vi "Set - TFA User Control Refs.vi"(0 "reference in":refnum<class "SPWB.lvclass">, 5 "error in (no error)":errorcluster, 7 "TFA User Control Refs":T1) -> (14 "reference out":refnum<class "SPWB.lvclass">, 19 "error out":errorcluster)   [LabVIEW 2022 SP3, in "SPWB.lvclass"]
uses:
  SPWB.lvclass
  controls/TFA - User Control References.ctl
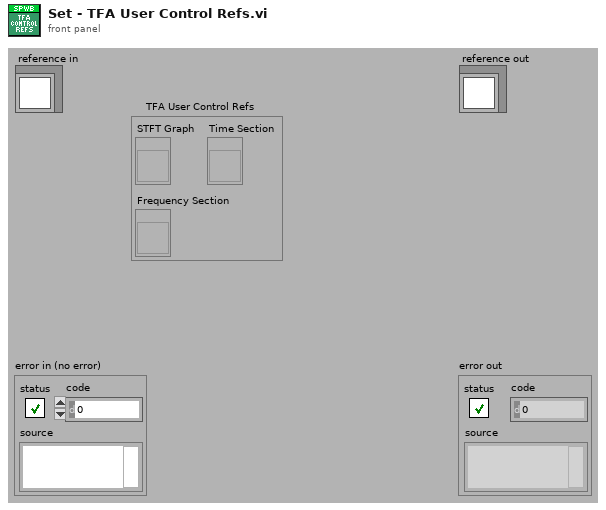
[diagram p1: front panel]
types:
  T1 = typedef "SPWB.lvclass/TFA - User Control References.ctl" = cluster{"STFT Graph":refnum<vi>, "Time Section":refnum<vi>, "Frequency Section":refnum<vi>}
  T2 = typedef "SPWB.lvclass/ObjectAttributesRef.ctl" = refnum<data-value>
  T3 = typedef "SPWB.lvclass/ObjectAttributes.ctl" = cluster{"Window Name Index":string, "Data":refnum<class "GSwFormDSP.lvclass">, "Registration":refnum<class "Registration.lvclass">, "TFA User Control Refs ":T1}
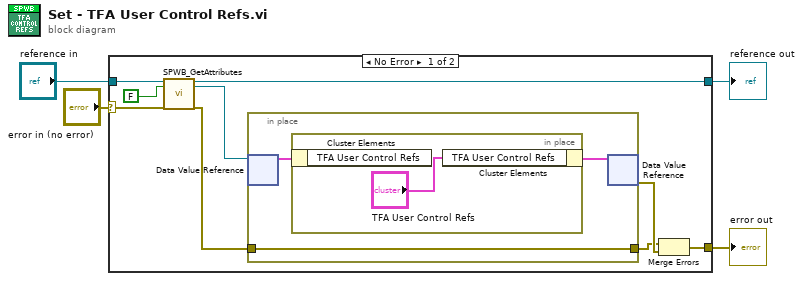
[diagram p0: block diagram]
diagram:
  n1 = case shown="No Error" "error in (no error)" {
    selector: "error in (no error)" -> [w8 w19]
    tunnel: [w13 w19] -> w3
    tunnel: [w6 w18] -> w1
    tunnel: "reference in" -> [w10 w18]
    frame No Error {
      n2 = call "SPWB_GetAttributes.vi"("reference in"=w10, "return data? (T)"=FALSE, "error in (no error)"=w8) -> ("reference out"=w6:refnum<class "SPWB.lvclass">, "attributes ref"=w5:T2, "error out"=w7:errorcluster)  [unwired: 13 in, 1 out]
      n3 = in-place {
        in-place-border: w7 -> [w14]
        in-place-border: [w14] -> w11
        n4 = in-place-dvr #1(w5) -> (w15:T3)  [unwired: 1 out]
        n5 = in-place {
          n6 = in-place-cluster #2(w15) -> ()  [unwired: 1 out]
          n7 = in-place-cluster #2("TFA User Control Refs"="TFA User Control Refs") -> (w16:T3)
        }
        n8 = in-place-dvr #1(w16) -> (w12:errorcluster)  [unwired: 1 out]
      }
      n9 = Merge Errors(w11, w12) -> (w13:errorcluster)
    }
    frame Error {
    }
  }
  "error out" <- w3
  "reference out" <- w1
